vi "Build.vi"   [LabVIEW 2018, in "Scripts.lvlib"]
uses:
  Scripts.lvlib
  <vilib>/Field R&D Services/Labricator/Toolkit/Field_RnD_Services_Labricator_Toolkit.lvlib
panel:
  # "Overview: Builds all Source Distribution specifications for this project\nRequirements: LabVIEW 2015 or newer, Labricator Development Kit, HTML Help Workshop\nInstructions: Run this VI.\n\nThis VI builds all of the build specifications for this project. Any version of LabVIEW that supports projects and the Application Builder API can be used."
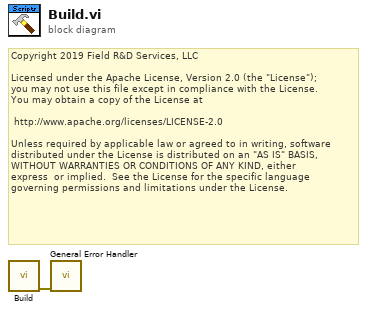
[diagram p0: block diagram]
diagram:
  # "Copyright 2019 Field R&D Services, LLC\n\nLicensed under the Apache License, Version 2.0 (the \"License\");\nyou may not use this file except in compliance with the License.\nYou may obtain a copy of the License at\n\n\thttp://www.apache.org/licenses/LICENSE-2.0\n\nUnless required by applicable law or agreed to in writing, software\ndistributed under the License is distributed on an \"AS IS\" BASIS,\nWITHOUT WARRANTIES OR CONDITIONS OF ANY KIND, either \nexpress  or implied.  See the License for the specific language \ngoverning permissions and limitations under the License."
  n1 = call <vilib>:"Build.vi"() -> ("Error Out"=w1:errorcluster)  [unwired: 11 in]
  n2 = call <vilib>:"General Error Handler.vi"("error in (no error)"=w1) -> ()  [unwired: 10 in, 5 out]
